vi "GeoData.vi"() -> ()   [LabVIEW 2017] (continued)
County\tH1\n69334\t31157\tBayard\tNE\tScotts Bluff County\tH1\n69341\t31157\tGering\tNE\tScotts Bluff County\tH1\n68428\t31159\tRaymond\tNE\tSeward County\tH1\n68460\t31159\tWaco\tNE\tSeward County\tH1\n68364\t31159\tGoehner\tNE\tSeward County\tH1\n68434\t31159\tSeward\tNE\tSeward County\tH1\n68367\t31159\tGresham\tNE\tSeward County\tH1\n68339\t31159\tDenton\tNE\tSeward County\tH1\n68360\t31159\tGarland\tNE\tSeward County\tH1\n68065\t31159\tValparaiso\tNE\tSeward County\tH1\n68423\t31159\tPleasant dale\tNE\tSeward County\tH1\n68528\t31159\tLincoln\tNE\tSeward County\tH1\n68343\t31159\tDorchester\tNE\tSeward County\tH1\n68669\t31159\tUlysses\tNE\tSeward County\tH1\n68314\t31159\tBee\tNE\tSeward County\tH1\n68359\t31159\tFriend\tNE\tSeward County\tH1\n68439\t31159\tStaplehurst\tNE\tSeward County\tH1\n68313\t31159\tBeaver crossing\tNE\tSeward County\tH1\n68405\t31159\tMilford\tNE\tSeward County\tH1\n68456\t31159\tUtica\tNE\tSeward County\tH1\n68330\t31159\tCordova\tNE\tSeward County\tH1\n69343\t31161\tGordon\tNE\tSheridan County\tH1\n69351\t31161\tLakeside\tNE\tSheridan County\tH1\n69301\t31161\tAlliance\tNE\tSheridan County\tH1\n69360\t31161\tRushville\tNE\tSheridan County\tH1\n69335\t31161\tBingham\tNE\tSheridan County\tH1\n69337\t31161\tChadron\tNE\tSheridan County\tH1\n69347\t31161\tHay springs\tNE\tSheridan County\tH1\n69333\t31161\tAshby\tNE\tSheridan County\tH1\n69340\t31161\tEllsworth\tNE\tSheridan County\tH1\n69365\t31161\tWhiteclay\tNE\tSheridan County\tH1\n68844\t31163\tHazard\tNE\tSherman County\tH1\n68815\t31163\tArcadia\tNE\tSherman County\tH1\n68817\t31163\tAshton\tNE\tSherman County\tH1\n68859\t31163\tNorth loup\tNE\tSherman County\tH1\n68852\t31163\tLitchfield\tNE\tSherman County\tH1\n68869\t31163\tRavenna\tNE\tSherman County\tH1\n68853\t31163\tLoup city\tNE\tSherman County\tH1\n68871\t31163\tRockville\tNE\tSherman County\tH1\n68820\t31163\tBoelus\tNE\tSherman County\tH1\n69358\t31165\tMorrill\tNE\tSioux County\tH1\n69301\t31165\tAlliance\tNE\tSioux County\tH1\n69357\t31165\tMitchell\tNE\tSioux County\tH1\n69348\t31165\tHemingford\tNE\tSioux County\tH1\n69346\t31165\tHarrison\tNE\tSioux County\tH1\n69361\t31165\tScottsbluff\tNE\tSioux County\tH1\n69339\t31165\tCrawford\tNE\tSioux County\tH1\n69356\t31165\tMinatare\tNE\tSioux County\tH1\n69354\t31165\tMarsland\tNE\tSioux County\tH1\n68779\t31167\tStanton\tNE\tStanton County\tH1\n68748\t31167\tMadison\tNE\tStanton County\tH1\n68641\t31167\tHowells\tNE\tStanton County\tH1\n68701\t31167\tNorfolk\tNE\tStanton County\tH1\n68740\t31167\tHoskins\tNE\tStanton County\tH1\n68768\t31167\tPilger\tNE\tStanton County\tH1\n68643\t31167\tLeigh\tNE\tStanton County\tH1\n68631\t31167\tCreston\tNE\tStanton County\tH1\n68629\t31167\tClarkson\tNE\tStanton County\tH1\n68943\t31169\tHardy\tNE\tThayer County\tH1\n68340\t31169\tDeshler\tNE\tThayer County\tH1\n68303\t31169\tAlexandria\tNE\tThayer County\tH1\n68429\t31169\tReynolds\tNE\tThayer County\tH1\n68326\t31169\tCarleton\tNE\tThayer County\tH1\n68325\t31169\tByron\tNE\tThayer County\tH1\n68327\t31169\tChester\tNE\tThayer County\tH1\n68315\t31169\tBelvidere\tNE\tThayer County\tH1\n68974\t31169\tRuskin\tNE\tThayer County\tH1\n68964\t31169\tOak\tNE\tThayer County\tH1\n68370\t31169\tHebron\tNE\tThayer County\tH1\n68375\t31169\tHubbell\tNE\tThayer County\tH1\n68322\t31169\tBruning\tNE\tThayer County\tH1\n68362\t31169\tGilead\tNE\tThayer County\tH1\n68335\t31169\tDavenport\tNE\tThayer County\tH1\n69166\t31171\tThedford\tNE\tThomas County\tH1\n69157\t31171\tPurdum\tNE\tThomas County\tH1\n69161\t31171\tSeneca\tNE\tThomas County\tH1\n69163\t31171\tStapleton\tNE\tThomas County\tH1\n69142\t31171\tHalsey\tNE\tThomas County\tH1\n68039\t31173\tMacy\tNE\tThurston County\tH1\n68047\t31173\tPender\tNE\tThurston County\tH1\n68062\t31173\tThurston\tNE\tThurston County\tH1\n68004\t31173\tBancroft\tNE\tThurston County\tH1\n68067\t31173\tWalthill\tNE\tThurston County\tH1\n68733\t31173\tEmerson\tNE\tThurston County\tH1\n68055\t31173\tRosalie\tNE\tThurston County\tH1\n68038\t31173\tLyons\tNE\tThurston County\tH1\n68020\t31173\tDecatur\tNE\tThurston County\tH1\n68784\t31173\tWakefield\tNE\tThurston County\tH1\n68071\t31173\tWinnebago\tNE\tThurston County\tH1\n68815\t31175\tArcadia\tNE\tValley County\tH1\n68837\t31175\tElyria\tNE\tValley County\tH1\n68862\t31175\tOrd\tNE\tValley County\tH1\n68823\t31175\tBurwell\tNE\tValley County\tH1\n68637\t31175\tEricson\tNE\tValley County\tH1\n68859\t31175\tNorth loup\tNE\tValley County\tH1\n68828\t31175\tComstock\tNE\tValley County\tH1\n68029\t31177\tHerman\tNE\tWashington County\tH1\n68152\t31177\tOmaha\tNE\tWashington County\tH1\n68007\t31177\tBennington\tNE\tWashington County\tH1\n68044\t31177\tNickerson\tNE\tWashington County\tH1\n68112\t31177\tOmaha\tNE\tWashington County\tH1\n68034\t31177\tKennard\tNE\tWashington County\tH1\n68023\t31177\tFort calhoun\tNE\tWashington County\tH1\n68122\t31177\tOmaha\tNE\tWashington County\tH1\n68064\t31177\tValley\tNE\tWashington County\tH1\n68008\t31177\tBlair\tNE\tWashington County\tH1\n68002\t31177\tArlington\tNE\tWashington County\tH1\n68025\t31177\tFremont\tNE\tWashington County\tH1\n68068\t31177\tWashington\tNE\tWashington County\tH1\n68031\t31177\tHooper\tNE\tWashington County\tH1\n68142\t31177\tOmaha\tNE\tWashington County\tH1\n68745\t31179\tLaurel\tNE\tWayne County\tH1\n68790\t31179\tWinside\tNE\tWayne County\tH1\n68047\t31179\tPender\tNE\tWayne County\tH1\n68701\t31179\tNorfolk\tNE\tWayne County\tH1\n68733\t31179\tEmerson\tNE\tWayne County\tH1\n68740\t31179\tHoskins\tNE\tWayne County\tH1\n68768\t31179\tPilger\tNE\tWayne County\tH1\n68723\t31179\tCarroll\tNE\tWayne County\tH1\n68787\t31179\tWayne\tNE\tWayne County\tH1\n68771\t31179\tRandolph\tNE\tWayne County\tH1\n68791\t31179\tWisner\tNE\tWayne County\tH1\n68784\t31179\tWakefield\tNE\tWayne County\tH1\n68957\t31181\tLawrence\tNE\tWebster County\tH1\n68928\t31181\tBladen\tNE\tWebster County\tH1\n68930\t31181\tBlue hill\tNE\tWebster County\tH1\n68942\t31181\tGuide rock\tNE\tWebster County\tH1\n68970\t31181\tRed cloud\tNE\tWebster County\tH1\n68932\t31181\tCampbell\tNE\tWebster County\tH1\n68952\t31181\tInavale\tNE\tWebster County\tH1\n68665\t31183\tSpalding\tNE\tWheeler County\tH1\n68725\t31183\tChambers\tNE\tWheeler County\tH1\n68637\t31183\tEricson\tNE\tWheeler County\tH1\n68636\t31183\tElgin\tNE\tWheeler County\tH1\n68735\t31183\tEwing\tNE\tWheeler County\tH1\n68622\t31183\tBartlett\tNE\tWheeler County\tH1\n68654\t31185\tPolk\tNE\tYork County\tH1\n68467\t31185\tYork\tNE\tYork County\tH1\n68460\t31185\tWaco\tNE\tYork County\tH1\n68367\t31185\tGresham\tNE\tYork County\tH1\n68401\t31185\tMc cool junction\tNE\tYork County\tH1\n68371\t31185\tHenderson\tNE\tYork County\tH1\n68316\t31185\tBenedict\tNE\tYork County\tH1\n68666\t31185\tStromsburg\tNE\tYork County\tH1\n68351\t31185\tExeter\tNE\tYork County\tH1\n68354\t31185\tFairmont\tNE\tYork County\tH1\n68319\t31185\tBradshaw\tNE\tYork County\tH1\n68979\t31185\tSutton\tNE\tYork County\tH1\n68365\t31185\tGrafton\tNE\tYork County\tH1\n68843\t31185\tHampton\tNE\tYork County\tH1\n89407\t32001\tFallon\tNV\tChurchill County\tH1\n89406\t32001\tFallon\tNV\tChurchill County\tH1\n89408\t32001\tFernley\tNV\tChurchill County\tH1\n89496\t32001\tFallon\tNV\tChurchill County\tH1\n89014\t32003\tHenderson\tNV\tClark County\tH1\n89012\t32003\tHenderson\tNV\tClark County\tH1\n89102\t32003\tLas vegas\tNV\tClark County\tH1\n89117\t32003\tLas vegas\tNV\tClark County\tH1\n89103\t32003\tLas vegas\tNV\tClark County\tH1\n89149\t32003\tLas vegas\tNV\tClark County\tH1\n89129\t32003\tLas vegas\tNV\tClark County\tH1\n89146\t32003\tLas vegas\tNV\tClark County\tH1\n89126\t32003\tLas vegas\tNV\tClark County\tH1\n89134\t32003\tLas vegas\tNV\tClark County\tH1\n89127\t32003\tLas vegas\tNV\tClark County\tH1\n89191\t32003\tNellis afb\tNV\tClark County\tH1\n89112\t32003\tLas vegas\tNV\tClark County\tH1\n89111\t32003\tLas vegas\tNV\tClark County\tH1\n89037\t32003\tCoyote springs\tNV\tClark County\tH1\n89030\t32003\tNorth las vegas\tNV\tClark County\tH1\n89029\t32003\tLaughlin\tNV\tClark County\tH1\n89109\t32003\tLas vegas\tNV\tClark County\tH1\n89084\t32003\tNorth las vegas\tNV\tClark County\tH1\n89114\t32003\tLas vegas\tNV\tClark County\tH1\n89120\t32003\tLas vegas\tNV\tClark County\tH1\n89141\t32003\tLas vegas\tNV\tClark County\tH1\n89158\t32003\tLas vegas\tNV\tClark County\tH1\n89170\t32003\tLas vegas\tNV\tClark County\tH1\n89157\t32003\tLas vegas\tNV\tClark County\tH1\n89151\t32003\tLas vegas\tNV\tClark County\tH1\n89024\t32003\tMesquite\tNV\tClark County\tH1\n89104\t32003\tLas vegas\tNV\tClark County\tH1\n89115\t32003\tLas vegas\tNV\tClark County\tH1\n89052\t32003\tHenderson\tNV\tClark County\tH1\n89148\t32003\tLas vegas\tNV\tClark County\tH1\n89169\t32003\tLas vegas\tNV\tClark County\tH1\n89138\t32003\tLas vegas\tNV\tClark County\tH1\n89180\t32003\tLas vegas\tNV\tClark County\tH1\n89130\t32003\tLas vegas\tNV\tClark County\tH1\n89086\t32003\tNorth las vegas\tNV\tClark County\tH1\n89016\t32003\tHenderson\tNV\tClark County\tH1\n89007\t32003\tBunkerville\tNV\tClark County\tH1\n89155\t32003\tLas vegas\tNV\tClark County\tH1\n89087\t32003\tNorth las vegas\tNV\tClark County\tH1\n89153\t32003\tLas vegas\tNV\tClark County\tH1\n89006\t32003\tBoulder city\tNV\tClark County\tH1\n89027\t32003\tMesquite\tNV\tClark County\tH1\n89034\t32003\tMesquite\tNV\tClark County\tH1\n89101\t32003\tLas vegas\tNV\tClark County\tH1\n89106\t32003\tLas vegas\tNV\tClark County\tH1\n89160\t32003\tLas vegas\tNV\tClark County\tH1\n89166\t32003\tLas vegas\tNV\tClark County\tH1\n89025\t32003\tMoapa\tNV\tClark County\tH1\n89018\t32003\tIndian springs\tNV\tClark County\tH1\n89009\t32003\tHenderson\tNV\tClark County\tH1\n89125\t32003\tLas vegas\tNV\tClark County\tH1\n89195\t32003\tLas vegas\tNV\tClark County\tH1\n89002\t32003\tHenderson\tNV\tClark County\tH1\n89005\t32003\tBoulder city\tNV\tClark County\tH1\n89015\t32003\tHenderson\tNV\tClark County\tH1\n89028\t32003\tLaughlin\tNV\tClark County\tH1\n89033\t32003\tNorth las vegas\tNV\tClark County\tH1\n89021\t32003\tLogandale\tNV\tClark County\tH1\n89123\t32003\tLas vegas\tNV\tClark County\tH1\n89053\t32003\tHenderson\tNV\tClark County\tH1\n89145\t32003\tLas vegas\tNV\tClark County\tH1\n89143\t32003\tLas vegas\tNV\tClark County\tH1\n89183\t32003\tLas vegas\tNV\tClark County\tH1\n89137\t32003\tLas vegas\tNV\tClark County\tH1\n89124\t32003\tLas vegas\tNV\tClark County\tH1\n89162\t32003\tLas vegas\tNV\tClark County\tH1\n89039\t32003\tCal nev ari\tNV\tClark County\tH1\n89152\t32003\tLas vegas\tNV\tClark County\tH1\n89031\t32003\tNorth las vegas\tNV\tClark County\tH1\n89074\t32003\tHenderson\tNV\tClark County\tH1\n89121\t32003\tLas vegas\tNV\tClark County\tH1\n89122\t32003\tLas vegas\tNV\tClark County\tH1\n89054\t32003\tSloan\tNV\tClark County\tH1\n89147\t32003\tLas vegas\tNV\tClark County\tH1\n89131\t32003\tLas vegas\tNV\tClark County\tH1\n89128\t32003\tLas vegas\tNV\tClark County\tH1\n89178\t32003\tLas vegas\tNV\tClark County\tH1\n89173\t32003\tLas vegas\tNV\tClark County\tH1\n89179\t32003\tLas vegas\tNV\tClark County\tH1\n89161\t32003\tLas vegas\tNV\tClark County\tH1\n89132\t32003\tLas vegas\tNV\tClark County\tH1\n89046\t32003\tSearchlight\tNV\tClark County\tH1\n89165\t32003\tLas vegas\tNV\tClark County\tH1\n89154\t32003\tLas vegas\tNV\tClark County\tH1\n89004\t32003\tBlue diamond\tNV\tClark County\tH1\n89032\t32003\tNorth las vegas\tNV\tClark County\tH1\n89119\t32003\tLas vegas\tNV\tClark County\tH1\n89085\t32003\tNorth las vegas\tNV\tClark County\tH1\n89142\t32003\tLas vegas\tNV\tClark County\tH1\n89144\t32003\tLas vegas\tNV\tClark County\tH1\n89135\t32003\tLas vegas\tNV\tClark County\tH1\n89156\t32003\tLas vegas\tNV\tClark County\tH1\n89193\t32003\tLas vegas\tNV\tClark County\tH1\n89105\t32003\tLas vegas\tNV\tClark County\tH1\n89011\t32003\tHenderson\tNV\tClark County\tH1\n89019\t32003\tJean\tNV\tClark County\tH1\n89036\t32003\tNorth las vegas\tNV\tClark County\tH1\n89044\t32003\tHenderson\tNV\tClark County\tH1\n89108\t32003\tLas vegas\tNV\tClark County\tH1\n89110\t32003\tLas vegas\tNV\tClark County\tH1\n89113\t32003\tLas vegas\tNV\tClark County\tH1\n89118\t32003\tLas vegas\tNV\tClark County\tH1\n89107\t32003\tLas vegas\tNV\tClark County\tH1\n89081\t32003\tNorth las vegas\tNV\tClark County\tH1\n89077\t32003\tHenderson\tNV\tClark County\tH1\n89139\t32003\tLas vegas\tNV\tClark County\tH1\n89136\t32003\tLas vegas\tNV\tClark County\tH1\n89133\t32003\tLas vegas\tNV\tClark County\tH1\n89040\t32003\tOverton\tNV\tClark County\tH1\n89116\t32003\tLas vegas\tNV\tClark County\tH1\n89140\t32003\tLas vegas\tNV\tClark County\tH1\n89199\t32003\tLas vegas\tNV\tClark County\tH1\n89150\t32003\tLas vegas\tNV\tClark County\tH1\n89444\t32005\tWellington\tNV\tDouglas County\tH1\n89705\t32005\tCarson city\tNV\tDouglas County\tH1\n89449\t32005\tStateline\tNV\tDouglas County\tH1\n89413\t32005\tGlenbrook\tNV\tDouglas County\tH1\n89423\t32005\tMinden\tNV\tDouglas County\tH1\n89448\t32005\tZephyr cove\tNV\tDouglas County\tH1\n89411\t32005\tGenoa\tNV\tDouglas County\tH1\n89410\t32005\tGardnerville\tNV\tDouglas County\tH1\n89701\t32005\tCarson city\tNV\tDouglas County\tH1\n89460\t32005\tGardnerville\tNV\tDouglas County\tH1\n89821\t32007\tCrescent valley\tNV\tElko County\tH1\n89825\t32007\tJackpot\tNV\tElko County\tH1\n89883\t32007\tWest wendover\tNV\tElko County\tH1\n89828\t32007\tLamoille\tNV\tElko County\tH1\n89823\t32007\tDeeth\tNV\tElko County\tH1\n89830\t32007\tMontello\tNV\tElko County\tH1\n89801\t32007\tElko\tNV\tElko County\tH1\n89815\t32007\tSpring creek\tNV\tElko County\tH1\n89832\t32007\tOwyhee\tNV\tElko County\tH1\n89803\t32007\tElko\tNV\tElko County\tH1\n89834\t32007\tTuscarora\tNV\tElko County\tH1\n89835\t32007\tWells\tNV\tElko County\tH1\n89822\t32007\tCarlin\tNV\tElko County\tH1\n89833\t32007\tRuby valley\tNV\tElko County\tH1\n89831\t32007\tMountain city\tNV\tElko County\tH1\n89826\t32007\tJarbidge\tNV\tElko County\tH1\n89013\t32009\tGoldfield\tNV\tEsmeralda County\tH1\n89047\t32009\tSilverpeak\tNV\tEsmeralda County\tH1\n89010\t32009\tDyer\tNV\tEsmeralda County\tH1\n89821\t32011\tCrescent valley\tNV\tEureka County\tH1\n89820\t32011\tBattle mountain\tNV\tEureka County\tH1\n89316\t32011\tEureka\tNV\tEureka County\tH1\n89426\t32013\tParadise valley\tNV\tHumboldt County\tH1\n89445\t32013\tWinnemucca\tNV\tHumboldt County\tH1\n89425\t32013\tOrovada\tNV\tHumboldt County\tH1\n89414\t32013\tGolconda\tNV\tHumboldt County\tH1\n89421\t32013\tMc dermitt\tNV\tHumboldt County\tH1\n89438\t32013\tValmy\tNV\tHumboldt County\tH1\n89820\t32015\tBattle mountain\tNV\tLander County\tH1\n89310\t32015\tAustin\tNV\tLander County\tH1\n89042\t32017\tPanaca\tNV\tLincoln County\tH1\n89017\t32017\tHiko\tNV\tLincoln County\tH1\n89043\t32017\tPioche\tNV\tLincoln County\tH1\n89001\t32017\tAlamo\tNV\tLincoln County\tH1\n89008\t32017\tCaliente\tNV\tLincoln County\tH1\n89444\t32019\tWellington\tNV\tLyon County\tH1\n89447\t32019\tYerington\tNV\tLyon County\tH1\n89406\t32019\tFallon\tNV\tLyon County\tH1\n89408\t32019\tFernley\tNV\tLyon County\tH1\n89429\t32019\tSilver springs\tNV\tLyon County\tH1\n89428\t32019\tSilver city\tNV\tLyon County\tH1\n89430\t32019\tSmith\tNV\tLyon County\tH1\n89706\t32019\tCarson city\tNV\tLyon County\tH1\n89403\t32019\tDayton\tNV\tLyon County\tH1\n89415\t32021\tHawthorne\tNV\tMineral County\tH1\n89420\t32021\tLuning\tNV\tMineral County\tH1\n89422\t32021\tMina\tNV\tMineral County\tH1\n89427\t32021\tSchurz\tNV\tMineral County\tH1\n89041\t32023\tPahrump\tNV\tNye County\tH1\n89020\t32023\tAmargosa valley\tNV\tNye County\tH1\n89045\t32023\tRound mountain\tNV\tNye County\tH1\n89049\t32023\tTonopah\tNV\tNye County\tH1\n89003\t32023\tBeatty\tNV\tNye County\tH1\n89409\t32023\tGabbs\tNV\tNye County\tH1\n89023\t32023\tMercury\tNV\tNye County\tH1\n89061\t32023\tPahrump\tNV\tNye County\tH1\n89048\t32023\tPahrump\tNV\tNye County\tH1\n89060\t32023\tPahrump\tNV\tNye County\tH1\n89022\t32023\tManhattan\tNV\tNye County\tH1\n89445\t32027\tWinnemucca\tNV\tPershing County\tH1\n89418\t32027\tImlay\tNV\tPershing County\tH1\n89404\t32027\tDenio\tNV\tPershing County\tH1\n89419\t32027\tLovelock\tNV\tPershing County\tH1\n89434\t32029\tSparks\tNV\tStorey County\tH1\n89521\t32029\tReno\tNV\tStorey County\tH1\n89440\t32029\tVirginia city\tNV\tStorey County\tH1\n89403\t32029\tDayton\tNV\tStorey County\tH1\n89508\t32029\tReno\tNV\tStorey County\tH1\n89431\t32031\tSparks\tNV\tWashoe County\tH1\n89511\t32031\tReno\tNV\tWashoe County\tH1\n89523\t32031\tReno\tNV\tWashoe County\tH1\n89504\t32031\tReno\tNV\tWashoe County\tH1\n89412\t32031\tGerlach\tNV\tWashoe County\tH1\n89442\t32031\tWadsworth\tNV\tWashoe County\tH1\n89435\t32031\tSparks\tNV\tWashoe County\tH1\n89439\t32031\tVerdi\tNV\tWashoe County\tH1\n89432\t32031\tSparks\tNV\tWashoe County\tH1\n89434\t32031\tSparks\tNV\tWashoe County\tH1\n89521\t32031\tReno\tNV\tWashoe County\tH1\n89506\t32031\tReno\tNV\tWashoe County\tH1\n89570\t32031\tReno\tNV\tWashoe County\tH1\n89703\t32031\tCarson city\tNV\tWashoe County\tH1\n89501\t32031\tReno\tNV\tWashoe County\tH1\n89512\t32031\tReno\tNV\tWashoe County\tH1\n89451\t32031\tIncline village\tNV\tWashoe County\tH1\n89704\t32031\tWashoe valley\tNV\tWashoe County\tH1\n89424\t32031\tNixon\tNV\tWashoe County\tH1\n89436\t32031\tSparks\tNV\tWashoe County\tH1\n89519\t32031\tReno\tNV\tWashoe County\tH1\n89513\t32031\tReno\tNV\tWashoe County\tH1\n89507\t32031\tReno\tNV\tWashoe County\tH1\n89595\t32031\tReno\tNV\tWashoe County\tH1\n89599\t32031\tReno\tNV\tWashoe County\tH1\n89503\t32031\tReno\tNV\tWashoe County\tH1\n89402\t32031\tCrystal bay\tNV\tWashoe County\tH1\n89515\t32031\tReno\tNV\tWashoe County\tH1\n89557\t32031\tReno\tNV\tWashoe County\tH1\n89441\t32031\tSparks\tNV\tWashoe County\tH1\n89502\t32031\tReno\tNV\tWashoe County\tH1\n89450\t32031\tIncline village\tNV\tWashoe County\tH1\n89533\t32031\tReno\tNV\tWashoe County\tH1\n89433\t32031\tSun valley\tNV\tWashoe County\tH1\n89509\t32031\tReno\tNV\tWashoe County\tH1\n89510\t32031\tReno\tNV\tWashoe County\tH1\n89508\t32031\tReno\tNV\tWashoe County\tH1\n89505\t32031\tReno\tNV\tWashoe County\tH1\n89318\t32033\tMc gill\tNV\tWhite Pine County\tH1\n89317\t32033\tLund\tNV\tWhite Pine County\tH1\n89314\t32033\tDuckwater\tNV\tWhite Pine County\tH1\n89311\t32033\tBaker\tNV\tWhite Pine County\tH1\n89319\t32033\tRuth\tNV\tWhite Pine County\tH1\n89301\t32033\tEly\tNV\tWhite Pine County\tH1\n89705\t32510\tCarson city\tNV\tCarson City\tC7\n89712\t32510\tCarson city\tNV\tCarson City\tC7\n89713\t32510\tCarson city\tNV\tCarson City\tC7\n89423\t32510\tMinden\tNV\tCarson City\tC7\n89703\t32510\tCarson city\tNV\tCarson City\tC7\n89721\t32510\tCarson city\tNV\tCarson City\tC7\n89706\t32510\tCarson city\tNV\tCarson City\tC7\n89714\t32510\tCarson city\tNV\tCarson City\tC7\n89702\t32510\tCarson city\tNV\tCarson City\tC7\n89711\t32510\tCarson city\tNV\tCarson City\tC7\n89701\t32510\tCarson city\tNV\tCarson City\tC7\n3253\t33001\tMeredith\tNH\tBelknap County\tH1\n3218\t33001\tBarnstead\tNH\tBelknap County\tH1\n3245\t33001\tHolderness\tNH\tBelknap County\tH1\n3299\t33001\tTilton\tNH\tBelknap County\tH1\n3220\t33001\tBelmont\tNH\tBelknap County\tH1\n3217\t33001\tAshland\tNH\tBelknap County\tH1\n3256\t33001\tNew hampton\tNH\tBelknap County\tH1\n3837\t33001\tGilmanton iron works\tNH\tBelknap County\tH1\n3809\t33001\tAlton\tNH\tBelknap County\tH1\n3246\t33001\tLaconia\tNH\tBelknap County\tH1\n3254\t33001\tMoultonborough\tNH\tBelknap County\tH1\n3276\t33001\tTilton\tNH\tBelknap County\tH1\n3289\t33001\tWinnisquam\tNH\tBelknap County\tH1\n3252\t33001\tLochmere\tNH\tBelknap County\tH1\n3249\t33001\tGilford\tNH\tBelknap County\tH1\n3226\t33001\tCenter harbor\tNH\tBelknap County\tH1\n3810\t33001\tAlton bay\tNH\tBelknap County\tH1\n3225\t33001\tCenter barnstead\tNH\tBelknap County\tH1\n3237\t33001\tGilmanton\tNH\tBelknap County\tH1\n3269\t33001\tSanbornton\tNH\tBelknap County\tH1\n3838\t33003\tGlen\tNH\tCarroll County\tH1\n3886\t33003\tTamworth\tNH\tCarroll County\tH1\n3847\t33003\tKearsarge\tNH\tCarroll County\tH1\n3882\t33003\tEffingham\tNH\tCarroll County\tH1\n3864\t33003\tOssipee\tNH\tCarroll County\tH1\n3850\t33003\tMelvin village\tNH\tCarroll County\tH1\n3836\t33003\tFreedom\tNH\tCarroll County\tH1\n3812\t33003\tBartlett\tNH\tCarroll County\tH1\n3254\t33003\tMoultonborough\tNH\tCarroll County\tH1\n3849\t33003\tMadison\tNH\tCarroll County\tH1\n3887\t33003\tUnion\tNH\tCarroll County\tH1\n3227\t33003\tCenter sandwich\tNH\tCarroll County\tH1\n3845\t33003\tIntervale\tNH\tCarroll County\tH1\n3817\t33003\tChocorua\tNH\tCarroll County\tH1\n3897\t33003\tWonalancet\tNH\tCarroll County\tH1\n3814\t33003\tCenter ossipee\tNH\tCarroll County\tH1\n3894\t33003\tWolfeboro\tNH\tCarroll County\tH1\n3226\t33003\tCenter harbor\tNH\tCarroll County\tH1\n3818\t33003\tConway\tNH\tCarroll County\tH1\n3860\t33003\tNorth conway\tNH\tCarroll County\tH1\n3832\t33003\tEaton center\tNH\tCarroll County\tH1\n3830\t33003\tEast wakefield\tNH\tCarroll County\tH1\n3853\t33003\tMirror lake\tNH\tCarroll County\tH1\n3813\t33003\tCenter conway\tNH\tCarroll County\tH1\n3816\t33003\tCenter tuftonboro\tNH\tCarroll County\tH1\n3872\t33003\tSanbornville\tNH\tCarroll County\tH1\n3875\t33003\tSilver lake\tNH\tCarroll County\tH1\n3890\t33003\tWest ossipee\tNH\tCarroll County\tH1\n3883\t33003\tSouth tamworth\tNH\tCarroll County\tH1\n3896\t33003\tWolfeboro falls\tNH\tCarroll County\tH1\n3846\t33003\tJackson\tNH\tCarroll County\tH1\n3259\t33003\tNorth sandwich\tNH\tCarroll County\tH1\n3431\t33005\tKeene\tNH\tCheshire County\tH1\n3602\t33005\tAlstead\tNH\tCheshire County\tH1\n3467\t33005\tWestmoreland\tNH\tCheshire County\tH1\n3469\t33005\tWest swanzey\tNH\tCheshire County\tH1\n3451\t33005\tHinsdale\tNH\tCheshire County\tH1\n3447\t33005\tFitzwilliam\tNH\tCheshire County\tH1\n3456\t33005\tMarlow\tNH\tCheshire County\tH1\n3446\t33005\tSwanzey\tNH\tCheshire County\tH1\n3462\t33005\tSpofford\tNH\tCheshire County\tH1\n3466\t33005\tWest chesterfield\tNH\tCheshire County\tH1\n3435\t33005\tKeene\tNH\tCheshire County\tH1\n3464\t33005\tStoddard\tNH\tCheshire County\tH1\n3604\t33005\tDrewsville\tNH\tCheshire County\tH1\n3443\t33005\tChesterfield\tNH\tCheshire County\tH1\n3461\t33005\tRindge\tNH\tCheshire County\tH1\n3609\t33005\tNorth walpole\tNH\tCheshire County\tH1\n3450\t33005\tHarrisville\tNH\tCheshire County\tH1\n3457\t33005\tNelson\tNH\tCheshire County\tH1\n3452\t33005\tJaffrey\tNH\tCheshire County\tH1\n3470\t33005\tWinchester\tNH\tCheshire County\tH1\n3608\t33005\tWalpole\tNH\tCheshire County\tH1\n3465\t33005\tTroy\tNH\tCheshire County\tH1\n3455\t33005\tMarlborough\tNH\tCheshire County\tH1\n3458\t33005\tPeterborough\tNH\tCheshire County\tH1\n3280\t33005\tWashington\tNH\tCheshire County\tH1\n3441\t33005\tAshuelot\tNH\tCheshire County\tH1\n3444\t33005\tDublin\tNH\tCheshire County\tH1\n3445\t33005\tSullivan\tNH\tCheshire County\tH1\n3448\t33005\tGilsum\tNH\tCheshire County\tH1\n3593\t33007\tRandolph\tNH\tCoos County\tH1\n3592\t33007\tPittsburg\tNH\tCoos County\tH1\n3583\t33007\tJefferson\tNH\tCoos County\tH1\n3588\t33007\tMilan\tNH\tCoos County\tH1\n3574\t33007\tBethlehem\tNH\tCoos County\tH1\n3582\t33007\tGroveton\tNH\tCoos County\tH1\n3570\t33007\tBerlin\tNH\tCoos County\tH1\n3576\t33007\tColebrook\tNH\tCoos County\tH1\n3579\t33007\tErrol\tNH\tCoos County\tH1\n3589\t33007\tMount washington\tNH\tCoos County\tH1\n3595\t33007\tTwin mountain\tNH\tCoos County\tH1\n3598\t33007\tWhitefield\tNH\tCoos County\tH1\n3581\t33007\tGorham\tNH\tCoos County\tH1\n3584\t33007\tLancaster\tNH\tCoos County\tH1\n3590\t33007\tNorth stratford\tNH\tCoos County\tH1\n3575\t33007\tBretton woods\tNH\tCoos County\tH1\n3597\t33007\tWest stewartstown\tNH\tCoos County\tH1\n3245\t33009\tHolderness\tNH\tGrafton County\tH1\n3282\t33009\tWentworth\tNH\tGrafton County\tH1\n3774\t33009\tNorth haverhill\tNH\tGrafton County\tH1\n3784\t33009\tWest lebanon\tNH\tGrafton County\tH1\n3748\t33009\tEnfield\tNH\tGrafton County\tH1\n3215\t33009\tWaterville valley\tNH\tGrafton County\tH1\n3780\t33009\tPike\tNH\tGrafton County\tH1\n3217\t33009\tAshland\tNH\tGrafton County\tH1\n3750\t33009\tEtna\tNH\tGrafton County\tH1\n3240\t33009\tGrafton\tNH\tGrafton County\tH1\n3585\t33009\tLisbon\tNH\tGrafton County\tH1\n3238\t33009\tGlencliff\tNH\tGrafton County\tH1\n3222\t33009\tBristol\tNH\tGrafton County\tH1\n3251\t33009\tLincoln\tNH\tGrafton County\tH1\n3241\t33009\tHebron\tNH\tGrafton County\tH1\n3262\t33009\tNorth woodstock\tNH\tGrafton County\tH1\n3264\t33009\tPlymouth\tNH\tGrafton County\tH1\n3574\t33009\tBethlehem\tNH\tGrafton County\tH1\n3785\t33009\tWoodsville\tNH\tGrafton County\tH1\n3779\t33009\tPiermont\tNH\tGrafton County\tH1\n3766\t33009\tLebanon\tNH\tGrafton County\tH1\n3740\t33009\tBath\tNH\tGrafton County\tH1\n3580\t33009\tFranconia\tNH\tGrafton County\tH1\n3279\t33009\tWarren\tNH\tGrafton County\tH1\n3266\t33009\tRumney\tNH\tGrafton County\tH1\n3285\t33009\tThornton\tNH\tGrafton County\tH1\n3741\t33009\tCanaan\tNH\tGrafton County\tH1\n3768\t33009\tLyme\tNH\tGrafton County\tH1\n3771\t33009\tMonroe\tNH\tGrafton County\tH1\n3753\t33009\tGrantham\tNH\tGrafton County\tH1\n3756\t33009\tLebanon\tNH\tGrafton County\tH1\n3769\t33009\tLyme center\tNH\tGrafton County\tH1\n3223\t33009\tCampton\tNH\tGrafton County\tH1\n3755\t33009\tHanover\tNH\tGrafton County\tH1\n3777\t33009\tOrford\tNH\tGrafton County\tH1\n3749\t33009\tEnfield center\tNH\tGrafton County\tH1\n3598\t33009\tWhitefield\tNH\tGrafton County\tH1\n3561\t33009\tLittleton\tNH\tGrafton County\tH1\n3586\t33009\tSugar hill\tNH\tGrafton County\tH1\n3243\t33009\tHill\tNH\tGrafton County\tH1\n3765\t33009\tHaverhill\tNH\tGrafton County\tH1\n3033\t33011\tBrookline\tNH\tHillsborough County\tH1\n3086\t33011\tWilton\tNH\tHillsborough County\tH1\n3108\t33011\tManchester\tNH\tHillsborough County\tH1\n3449\t33011\tHancock\tNH\tHillsborough County\tH1\n3051\t33011\tHudson\tNH\tHillsborough County\tH1\n3054\t33011\tMerrimack\tNH\tHillsborough County\tH1\n3062\t33011\tNashua\tNH\tHillsborough County\tH1\n3055\t33011\tMilford\tNH\tHillsborough County\tH1\n3045\t33011\tGoffstown\tNH\tHillsborough County\tH1\n3052\t33011\tLitchfield\tNH\tHillsborough County\tH1\n3049\t33011\tHollis\tNH\tHillsborough County\tH1\n3109\t33011\tManchester\tNH\tHillsborough County\tH1\n3101\t33011\tManchester\tNH\tHillsborough County\tH1\n3060\t33011\tNashua\tNH\tHillsborough County\tH1\n3064\t33011\tNashua\tNH\tHillsborough County\tH1\n3082\t33011\tLyndeborough\tNH\tHillsborough County\tH1\n3070\t33011\tNew boston\tNH\tHillsborough County\tH1\n3084\t33011\tTemple\tNH\tHillsborough County\tH1\n3057\t33011\tMont vernon\tNH\tHillsborough County\tH1\n3110\t33011\tBedford\tNH\tHillsborough County\tH1\n3111\t33011\tManchester\tNH\tHillsborough County\tH1\n3063\t33011\tNashua\tNH\tHillsborough County\tH1\n3244\t33011\tHillsborough\tNH\tHillsborough County\tH1\n3281\t33011\tWeare\tNH\tHillsborough County\tH1\n3103\t33011\tManchester\tNH\tHillsborough County\tH1\n3071\t33011\tNew ipswich\tNH\tHillsborough County\tH1\n3105\t33011\tManchester\tNH\tHillsborough County\tH1\n3043\t33011\tFrancestown\tNH\tHillsborough County\tH1\n3104\t33011\tManchester\tNH\tHillsborough County\tH1\n3102\t33011\tManchester\tNH\tHillsborough County\tH1\n3076\t33011\tPelham\tNH\tHillsborough County\tH1\n3452\t33011\tJaffrey\tNH\tHillsborough County\tH1\n3061\t33011\tNashua\tNH\tHillsborough County\tH1\n3031\t33011\tAmherst\tNH\tHillsborough County\tH1\n3106\t33011\tHooksett\tNH\tHillsborough County\tH1\n3458\t33011\tPeterborough\tNH\tHillsborough County\tH1\n3442\t33011\tBennington\tNH\tHillsborough County\tH1\n3280\t33011\tWashington\tNH\tHillsborough County\tH1\n3047\t33011\tGreenfield\tNH\tHillsborough County\tH1\n3440\t33011\tAntrim\tNH\tHillsborough County\tH1\n3048\t33011\tGreenville\tNH\tHillsborough County\tH1\n3468\t33011\tWest peterborough\tNH\tHillsborough County\tH1\n3303\t33013\tConcord\tNH\tMerrimack County\tH1\n3221\t33013\tBradford\tNH\tMerrimack County\tH1\n3045\t33013\tGoffstown\tNH\tMerrimack County\tH1\n3220\t33013\tBelmont\tNH\tMerrimack County\tH1\n3224\t33013\tCanterbury\tNH\tMerrimack County\tH1\n3229\t33013\tContoocook\tNH\tMerrimack County\tH1\n3046\t33013\tDunbarton\tNH\tMerrimack County\tH1\n3216\t33013\tAndover\tNH\tMerrimack County\tH1\n3233\t33013\tElkins\tNH\tMerrimack County\tH1\n3273\t33013\tSouth sutton\tNH\tMerrimack County\tH1\n3231\t33013\tEast andover\tNH\tMerrimack County\tH1\n3276\t33013\tTilton\tNH\tMerrimack County\tH1\n3301\t33013\tConcord\tNH\tMerrimack County\tH1\n3278\t33013\tWarner\tNH\tMerrimack County\tH1\n3287\t33013\tWilmot\tNH\tMerrimack County\tH1\n3258\t33013\tChichester\tNH\tMerrimack County\tH1\n3305\t33013\tConcord\tNH\tMerrimack County\tH1\n3257\t33013\tNew london\tNH\tMerrimack County\tH1\n3281\t33013\tWeare\tNH\tMerrimack County\tH1\n3034\t33013\tCandia\tNH\tMerrimack County\tH1\n3302\t33013\tConcord\tNH\tMerrimack County\tH1\n3260\t33013\tNorth sutton\tNH\tMerrimack County\tH1\n3263\t33013\tPittsfield\tNH\tMerrimack County\tH1\n3242\t33013\tHenniker\tNH\tMerrimack County\tH1\n3234\t33013\tEpsom\tNH\tMerrimack County\tH1\n3268\t33013\tSalisbury\tNH\tMerrimack County\tH1\n3104\t33013\tManchester\tNH\tMerrimack County\tH1\n3102\t33013\tManchester\tNH\tMerrimack County\tH1\n3235\t33013\tFranklin\tNH\tMerrimack County\tH1\n3304\t33013\tBow\tNH\tMerrimack County\tH1\n3272\t33013\tSouth newbury\tNH\tMerrimack County\tH1\n3106\t33013\tHooksett\tNH\tMerrimack County\tH1\n3230\t33013\tDanbury\tNH\tMerrimack County\tH1\n3237\t33013\tGilmanton\tNH\tMerrimack County\tH1\n3307\t33013\tLoudon\tNH\tMerrimack County\tH1\n3275\t33013\tSuncook\tNH\tMerrimack County\tH1\n3280\t33013\tWashington\tNH\tMerrimack County\tH1\n3255\t33013\tNewbury\tNH\tMerrimack County\tH1\n3243\t33013\tHill\tNH\tMerrimack County\tH1\n3044\t33015\tFremont\tNH\tRockingham County\tH1\n3825\t33015\tBarrington\tNH\tRockingham County\tH1\n3819\t33015\tDanville\tNH\tRockingham County\tH1\n3857\t33015\tNewmarket\tNH\tRockingham County\tH1\n3840\t33015\tGreenland\tNH\tRockingham County\tH1\n3291\t33015\tWest nottingham\tNH\tRockingham County\tH1\n3803\t33015\tPortsmouth\tNH\tRockingham County\tH1\n3042\t33015\tEpping\tNH\tRockingham County\tH1\n3036\t33015\tChester\tNH\tRockingham County\tH1\n3841\t33015\tHampstead\tNH\tRockingham County\tH1\n3848\t33015\tKingston\tNH\tRockingham County\tH1\n3811\t33015\tAtkinson\tNH\tRockingham County\tH1\n3871\t33015\tRye beach\tNH\tRockingham County\tH1\n3032\t33015\tAuburn\tNH\tRockingham County\tH1\n3053\t33015\tLondonderry\tNH\tRockingham County\tH1\n3873\t33015\tSandown\tNH\tRockingham County\tH1\n3844\t33015\tHampton falls\tNH\tRockingham County\tH1\n3858\t33015\tNewton\tNH\tRockingham County\tH1\n3854\t33015\tNew castle\tNH\tRockingham County\tH1\n3862\t33015\tNorth hampton\tNH\tRockingham County\tH1\n3856\t33015\tNewfields\tNH\tRockingham County\tH1\n3041\t33015\tEast derry\tNH\tRockingham County\tH1\n3034\t33015\tCandia\tNH\tRockingham County\tH1\n3073\t33015\tNorth salem\tNH\tRockingham County\tH1\n3802\t33015\tPortsmouth\tNH\tRockingham County\tH1\n3103\t33015\tManchester\tNH\tRockingham County\tH1\n3263\t33015\tPittsfield\tNH\tRockingham County\tH1\n3234\t33015\tEpsom\tNH\tRockingham County\tH1\n3801\t33015\tPortsmouth\tNH\tRockingham County\tH1\n3827\t33015\tEast kingston\tNH\tRockingham County\tH1\n3885\t33015\tStratham\tNH\tRockingham County\tH1\n3874\t33015\tSeabrook\tNH\tRockingham County\tH1\n3104\t33015\tManchester\tNH\tRockingham County\tH1\n3079\t33015\tSalem\tNH\tRockingham County\tH1\n3842\t33015\tHampton\tNH\tRockingham County\tH1\n3826\t33015\tEast hampstead\tNH\tRockingham County\tH1\n3884\t33015\tStrafford\tNH\tRockingham County\tH1\n3865\t33015\tPlaistow\tNH\tRockingham County\tH1\n3037\t33015\tDeerfield\tNH\tRockingham County\tH1\n3038\t33015\tDerry\tNH\tRockingham County\tH1\n3077\t33015\tRaymond\tNH\tRockingham County\tH1\n3087\t33015\tWindham\tNH\tRockingham County\tH1\n3261\t33015\tNorthwood\tNH\tRockingham County\tH1\n3290\t33015\tNottingham\tNH\tRockingham County\tH1\n3824\t33015\tDurham\tNH\tRockingham County\tH1\n3833\t33015\tExeter\tNH\tRockingham County\tH1\n3843\t33015\tHampton\tNH\tRockingham County\tH1\n3870\t33015\tRye\tNH\tRockingham County\tH1\n3859\t33015\tNewton junction\tNH\tRockingham County\tH1\n3825\t33017\tBarrington\tNH\tStrafford County\tH1\n3839\t33017\tRochester\tNH\tStrafford County\tH1\n3857\t33017\tNewmarket\tNH\tStrafford County\tH1\n3878\t33017\tSomersworth\tNH\tStrafford County\tH1\n3042\t33017\tEpping\tNH\tStrafford County\tH1\n3809\t33017\tAlton\tNH\tStrafford County\tH1\n3867\t33017\tRochester\tNH\tStrafford County\tH1\n3815\t33017\tCenter strafford\tNH\tStrafford County\tH1\n3820\t33017\tDover\tNH\tStrafford County\tH1\n3851\t33017\tMilton\tNH\tStrafford County\tH1\n3887\t33017\tUnion\tNH\tStrafford County\tH1\n3868\t33017\tRochester\tNH\tStrafford County\tH1\n3852\t33017\tMilton mills\tNH\tStrafford County\tH1\n3861\t33017\tLee\tNH\tStrafford County\tH1\n3869\t33017\tRollinsford\tNH\tStrafford County\tH1\n3835\t33017\tFarmington\tNH\tStrafford County\tH1\n3855\t33017\tNew durham\tNH\tStrafford County\tH1\n3884\t33017\tStrafford\tNH\tStrafford County\tH1\n3823\t33017\tMadbury\tNH\tStrafford County\tH1\n3290\t33017\tNottingham\tNH\tStrafford County\tH1\n3824\t33017\tDurham\tNH\tStrafford County\tH1\n3821\t33017\tDover\tNH\tStrafford County\tH1\n3866\t33017\tRochester\tNH\tStrafford County\tH1\n3822\t33017\tDover\tNH\tStrafford County\tH1\n3748\t33019\tEnfield\tNH\tSullivan County\tH1\n3602\t33019\tAlstead\tNH\tSullivan County\tH1\n3605\t33019\tLempster\tNH\tSullivan County\tH1\n3607\t33019\tSouth acworth\tNH\tSullivan County\tH1\n3782\t33019\tSunapee\tNH\tSullivan County\tH1\n3781\t33019\tPlainfield\tNH\tSullivan County\tH1\n3770\t33019\tMeriden\tNH\tSullivan County\tH1\n3752\t33019\tGoshen\tNH\tSullivan County\tH1\n3284\t33019\tSpringfield\tNH\tSullivan County\tH1\n3601\t33019\tAcworth\tNH\tSullivan County\tH1\n3751\t33019\tGeorges mills\tNH\tSullivan County\tH1\n3745\t33019\tCornish\tNH\tSullivan County\tH1\n3257\t33019\tNew london\tNH\tSullivan County\tH1\n3244\t33019\tHillsborough\tNH\tSullivan County\tH1\n3773\t33019\tNewport\tNH\tSullivan County\tH1\n3753\t33019\tGrantham\tNH\tSullivan County\tH1\n3743\t33019\tClaremont\tNH\tSullivan County\tH1\n3603\t33019\tCharlestown\tNH\tSullivan County\tH1\n3746\t33019\tCornish flat\tNH\tSullivan County\tH1\n3280\t33019\tWashington\tNH\tSullivan County\tH1\n3754\t33019\tGuild\tNH\tSullivan County\tH1\n8225\t34001\tNorthfield\tNJ\tAtlantic County\tH1\n8326\t34001\tLandisville\tNJ\tAtlantic County\tH1\n8340\t34001\tMilmay\tNJ\tAtlantic County\tH1\n8405\t34001\tAtlantic city\tNJ\tAtlantic County\tH1\n8037\t34001\tHammonton\tNJ\tAtlantic County\tH1\n8270\t34001\tWoodbine\tNJ\tAtlantic County\tH1\n8361\t34001\tVineland\tNJ\tAtlantic County\tH1\n8203\t34001\tBrigantine\tNJ\tAtlantic County\tH1\n8232\t34001\tPleasantville\tNJ\tAtlantic County\tH1\n8201\t34001\tAbsecon\tNJ\tAtlantic County\tH1\n8401\t34001\tAtlantic city\tNJ\tAtlantic County\tH1\n8341\t34001\tMinotola\tNJ\tAtlantic County\tH1\n8217\t34001\tElwood\tNJ\tAtlantic County\tH1\n8094\t34001\tWilliamstown\tNJ\tAtlantic County\tH1\n8241\t34001\tPort republic\tNJ\tAtlantic County\tH1\n8215\t34001\tEgg harbor city\tNJ\tAtlantic County\tH1\n8360\t34001\tVineland\tNJ\tAtlantic County\tH1\n8346\t34001\tNewtonville\tNJ\tAtlantic County\tH1\n8342\t34001\tMizpah\tNJ\tAtlantic County\tH1\n8234\t34001\tEgg harbor township\tNJ\tAtlantic County\tH1\n8310\t34001\tBuena\tNJ\tAtlantic County\tH1\n8406\t34001\tVentnor city\tNJ\tAtlantic County\tH1\n8402\t34001\tMargate city\tNJ\tAtlantic County\tH1\n8317\t34001\tDorothy\tNJ\tAtlantic County\tH1\n8231\t34001\tOceanville\tNJ\tAtlantic County\tH1\n8220\t34001\tLeeds point\tNJ\tAtlantic County\tH1\n8205\t34001\tAbsecon\tNJ\tAtlantic County\tH1\n8244\t34001\tSomers point\tNJ\tAtlantic County\tH1\n8330\t34001\tMays landing\tNJ\tAtlantic County\tH1\n8319\t34001\tEstell manor\tNJ\tAtlantic County\tH1\n8350\t34001\tRichland\tNJ\tAtlantic County\tH1\n8213\t34001\tCologne\tNJ\tAtlantic County\tH1\n8221\t34001\tLinwood\tNJ\tAtlantic County\tH1\n8344\t34001\tNewfield\tNJ\tAtlantic County\tH1\n8403\t34001\tLongport\tNJ\tAtlantic County\tH1\n8404\t34001\tAtlantic city\tNJ\tAtlantic County\tH1\n8240\t34001\tPomona\tNJ\tAtlantic County\tH1\n7010\t34003\tCliffside park\tNJ\tBergen County\tH1\n7436\t34003\tOakland\tNJ\tBergen County\tH1\n7463\t34003\tWaldwick\tNJ\tBergen County\tH1\n7621\t34003\tBergenfield\tNJ\tBergen County\tH1\n7608\t34003\tTeterboro\tNJ\tBergen County\tH1\n7626\t34003\tCresskill\tNJ\tBergen County\tH1\n7666\t34003\tTeaneck\tNJ\tBergen County\tH1\n7660\t34003\tRidgefield park\tNJ\tBergen County\tH1\n7662\t34003\tRochelle park\tNJ\tBergen County\tH1\n7020\t34003\tEdgewater\tNJ\tBergen County\tH1\n7417\t34003\tFranklin lakes\tNJ\tBergen County\tH1\n7450\t34003\tRidgewood\tNJ\tBergen County\tH1\n7601\t34003\tHackensack\tNJ\tBergen County\tH1\n7648\t34003\tNorwood\tNJ\tBergen County\tH1\n7675\t34003\tWestwood\tNJ\tBergen County\tH1\n7073\t34003\tEast rutherford\tNJ\tBergen County\tH1\n7627\t34003\tDemarest\tNJ\tBergen County\tH1\n7653\t34003\tParamus\tNJ\tBergen County\tH1\n7495\t34003\tMahwah\tNJ\tBergen County\tH1\n7699\t34003\tTeterboro\tNJ\tBergen County\tH1\n7031\t34003\tNorth arlington\tNJ\tBergen County\tH1\n7047\t34003\tNorth bergen\tNJ\tBergen County\tH1\n7057\t34003\tWallington\tNJ\tBergen County\tH1\n7401\t34003\tAllendale\tNJ\tBergen County\tH1\n7407\t34003\tElmwood park\tNJ\tBergen County\tH1\n7506\t34003\tHawthorne\tNJ\tBergen County\tH1\n7481\t34003\tWyckoff\tNJ\tBergen County\tH1\n7630\t34003\tEmerson\tNJ\tBergen County\tH1\n7644\t34003\tLodi\tNJ\tBergen County\tH1\n7650\t34003\tPalisades park\tNJ\tBergen County\tH1\n7606\t34003\tSouth hackensack\tNJ\tBergen County\tH1\n7657\t34003\tRidgefield\tNJ\tBergen County\tH1\n7423\t34003\tHo ho kus\tNJ\tBergen County\tH1\n7024\t34003\tFort lee\tNJ\tBergen County\tH1\n7055\t34003\tPassaic\tNJ\tBergen County\tH1\n7071\t34003\tLyndhurst\tNJ\tBergen County\tH1\n7632\t34003\tEnglewood cliffs\tNJ\tBergen County\tH1\n7645\t34003\tMontvale\tNJ\tBergen County\tH1\n7641\t34003\tHaworth\tNJ\tBergen County\tH1\n7075\t34003\tWood ridge\tNJ\tBergen County\tH1\n7607\t34003\tMaywood\tNJ\tBergen County\tH1\n7647\t34003\tNorthvale\tNJ\tBergen County\tH1\n7620\t34003\tAlpine\tNJ\tBergen County\tH1\n7026\t34003\tGarfield\tNJ\tBergen County\tH1\n7032\t34003\tKearny\tNJ\tBergen County\tH1\n7070\t34003\tRutherford\tNJ\tBergen County\tH1\n7458\t34003\tSaddle river\tNJ\tBergen County\tH1\n7628\t34003\tDumont\tNJ\tBergen County\tH1\n7624\t34003\tCloster\tNJ\tBergen County\tH1\n7643\t34003\tLittle ferry\tNJ\tBergen County\tH1\n7022\t34003\tFairview\tNJ\tBergen County\tH1\n7072\t34003\tCarlstadt\tNJ\tBergen County\tH1\n7074\t34003\tMoonachie\tNJ\tBergen County\tH1\n7430\t34003\tMahwah\tNJ\tBergen County\tH1\n7452\t34003\tGlen rock\tNJ\tBergen County\tH1\n7446\t34003\tRamsey\tNJ\tBergen County\tH1\n7605\t34003\tLeonia\tNJ\tBergen County\tH1\n7631\t34003\tEnglewood\tNJ\tBergen County\tH1\n7649\t34003\tOradell\tNJ\tBergen County\tH1\n7604\t34003\tHasbrouck heights\tNJ\tBergen County\tH1\n7640\t34003\tHarrington park\tNJ\tBergen County\tH1\n7652\t34003\tParamus\tNJ\tBergen County\tH1\n7676\t34003\tTownship of washington\tNJ\tBergen County\tH1\n7670\t34003\tTenafly\tNJ\tBergen County\tH1\n7663\t34003\tSaddle brook\tNJ\tBergen County\tH1\n7451\t34003\tRidgewood\tNJ\tBergen County\tH1\n7410\t34003\tFair lawn\tNJ\tBergen County\tH1\n7603\t34003\tBogota\tNJ\tBergen County\tH1\n7646\t34003\tNew milford\tNJ\tBergen County\tH1\n7642\t34003\tHillsdale\tNJ\tBergen County\tH1\n7661\t34003\tRiver edge\tNJ\tBergen County\tH1\n7656\t34003\tPark ridge\tNJ\tBergen County\tH1\n7677\t34003\tWoodcliff lake\tNJ\tBergen County\tH1\n7432\t34003\tMidland park\tNJ\tBergen County\tH1\n7602\t34003\tHackensack\tNJ\tBergen County\tH1\n8036\t34005\tHainesport\tNJ\tBurlington County\tH1\n8505\t34005\tBordentown\tNJ\tBurlington County\tH1\n8501\t34005\tAllentown\tNJ\tBurlington County\tH1\n8610\t34005\tTrenton\tNJ\tBurlington County\tH1\n8019\t34005\tChatsworth\t
